vi "Main IU.vi"() -> ()   [LabVIEW 2019]
uses:
  <vilib>/Analysis/baseanly.llb/Mean (DBL).vi
  <vilib>/Analysis/NI_AALBase.lvlib
panel:
  out "Numeric":dbl
  in  "RESET 2":bool
  in  "Tiempo 2":dbl
  in  "Tiempo 1":dbl
  in  "Home":bool
  in  "Aceleración final Motor 2":dbl
  in  "Aceleración final Motor 1":dbl
  in  "Velocidad final Motor 2":dbl
  in  "Velocidad final Motor 1":dbl
  out "String":string
  in  "GO 2":bool
  in  "Aceleración inicial Motor 2":dbl
  in  "Aceleración inicial Motor 1":dbl
  in  "Velocidad inicial Motor 2":dbl
  in  "Velocidad inicial Motor 1":dbl
  in  "RESET 1":bool
  in  "Trayectoria":bool
  in  "GO":bool
  in  "Posición final Motor 2":dbl
  in  "MOTORES INDEPENDIENTES":bool
  in  "Tab Control":enum32{"Motor 1", "Motor 2"}(tab)
  out "Waveform Chart 6":waveform(dbl)[](graph)
  out "Waveform Chart 5":waveform(dbl)[](graph)
  out "Hall 1":bool
  out "Posición":waveform(dbl)[](graph)
  out "Hall 2":bool
  out "Waveform Chart 4":waveform(dbl)[](graph)
  out "Waveform Chart 3":waveform(dbl)[](graph)
  out "Hall 2":bool
  out "Waveform Chart 2":waveform(dbl)[](graph)
  out "Hall1":bool
  out "Saving Data":bool
  in  "Record Button":bool
  in  "Filename":path=path "test.lvm"
  in  "Stop UI and RT":bool
  in  "Stop UI":bool
  in  "Posición final motor 1":dbl
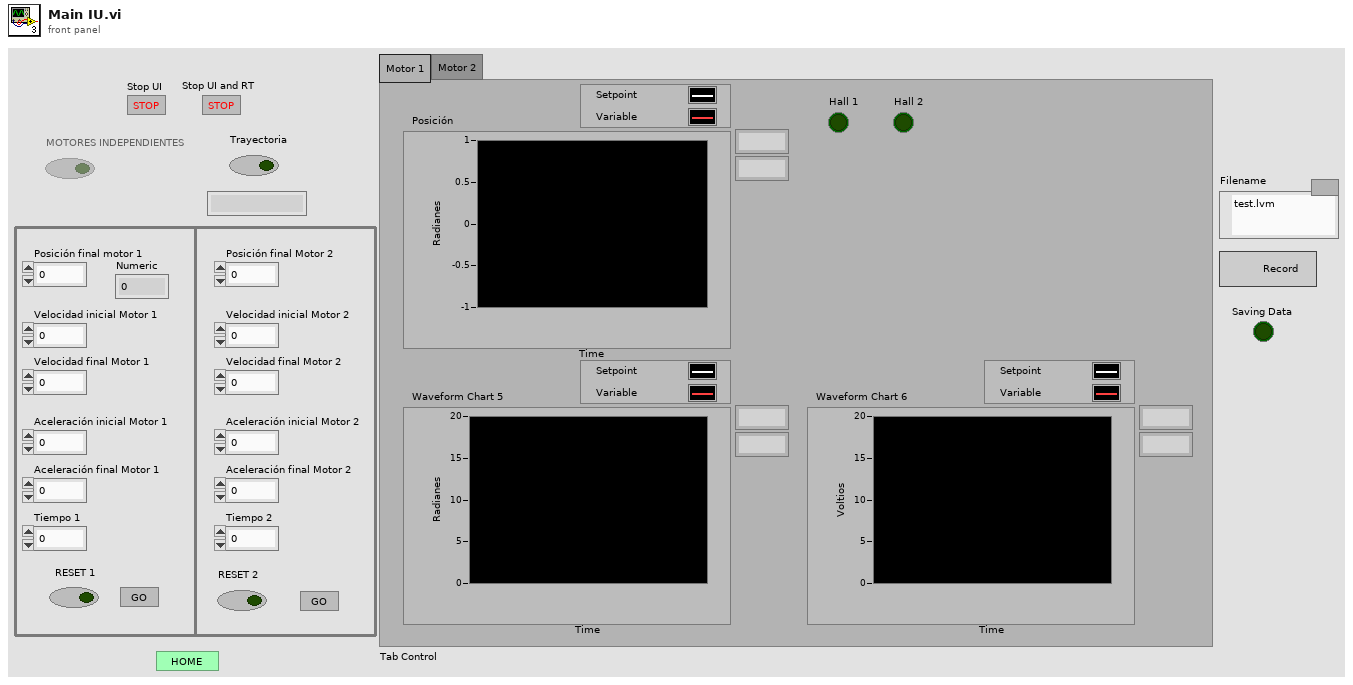
[diagram p1: front panel]
types:
  T1 = cluster{"Double":dbl, "dbl Scaled Value":dbl, "Output":dbl, "seconds since 1Jan1904":timestamp}
  T2 = cluster{"Double":dbl, "dbl Scaled Value":dbl, "Output":dbl, "seconds since 1Jan1904":timestamp}[]
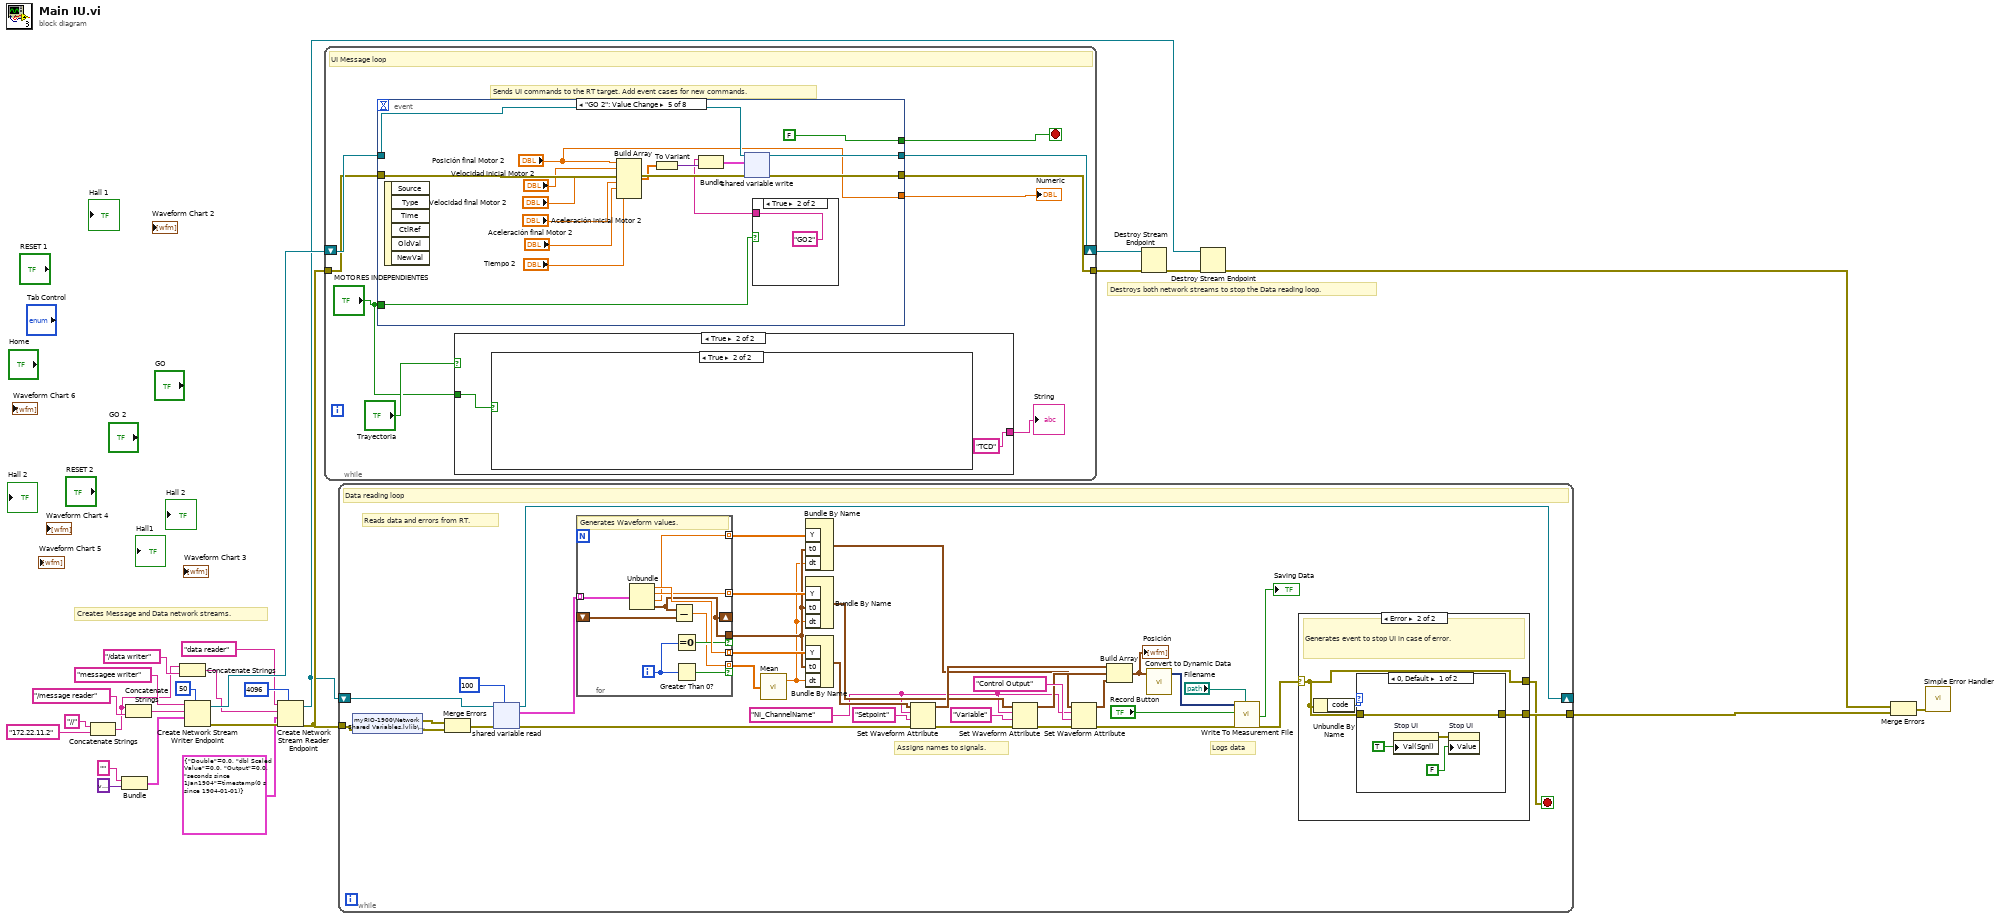
[diagram p0: block diagram]
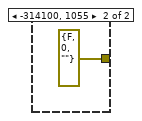
[diagram p3: hidden frame]
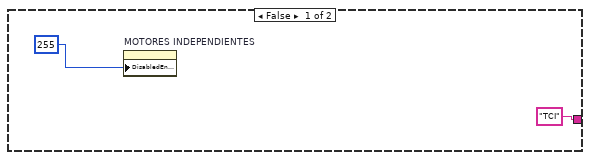
[diagram p4: hidden frame]
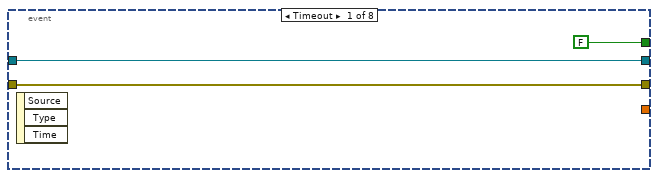
[diagram p6: hidden frame]
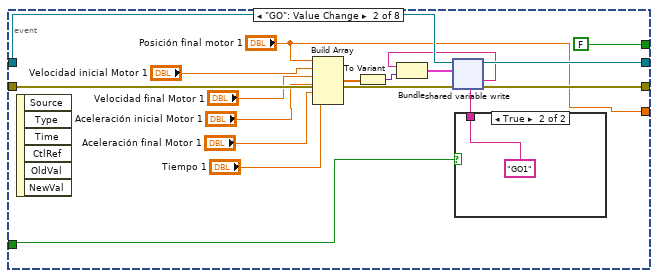
[diagram p7: hidden frame]
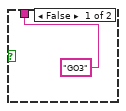
[diagram p8: hidden frame]
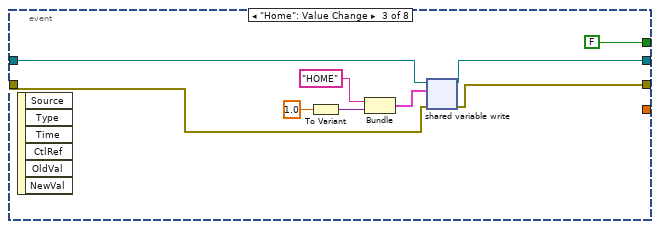
[diagram p9: hidden frame]
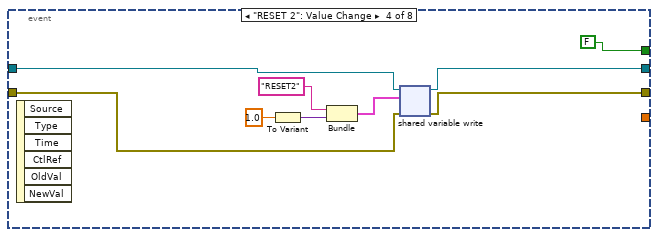
[diagram p10: hidden frame]
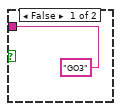
[diagram p11: hidden frame]
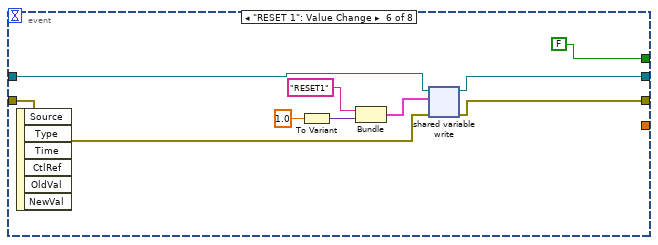
[diagram p12: hidden frame]
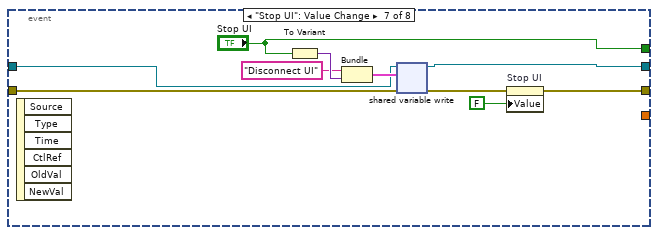
[diagram p13: hidden frame]
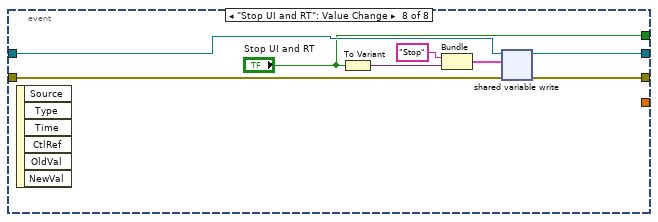
[diagram p14: hidden frame]
diagram:
  # "Destroys both network streams to stop the Data reading loop."
  # "Creates Message and Data network streams."
  n1 = Concatenate Strings("//", "172.22.11.2" ("myRIO IP")) -> (w1:string)
  n2 = Bundle("", variant) -> (w25:cluster{string, variant})  [unwired: 1 in]
  n3 = Concatenate Strings(w1, "/message reader") -> (w2:string)
  n4 = Concatenate Strings(w1, "/data writer") -> (w16:string)
  n5 = Create Network Stream Writer Endpoint(7:50 ("writer buffer size"), 9:w25, 10:w2, 11:"messagee writer" ("writer name")) -> (0:w13:errorcluster, 3:w19:refnum<k21>)  [unwired: 3 in]
  n6 = Create Network Stream Reader Endpoint(7:4096 ("reader buffer size"), 8:w13, 9:T1 {"Double"=0.0, "dbl Scaled Value"=0.0, "Output"=0.0, "seconds since 1Jan1904"=timestamp(0 s since 1904-01-01)} ("Data"), 10:w16, 11:"data reader" ("reader name")) -> (0:w12:errorcluster, 3:w5:refnum<k21>)  [unwired: 2 in]
  n7 = while {
    tunnel: w12 -> [w33]
    shift-right: [w32] -> w7
    shift-left: w19 -> [w34]
    tunnel: [w31] -> w8
    stop <- w30 stop-if-true
    # "Sends UI commands to the RT target. Add event cases for new commands."
    # "UI Message loop"
    n8 = event shown="[4] \"GO 2\": Value Change" {
      selector: _ -> [_ _ _ _ _ _ _ _]
      dyn-events: _ -> [_ _ _ _ _ _ _ _]
      timeout: _ -> [_ _ _ _ _ _ _ _]
      tunnel: w34 -> [w41 w57 w65 w71 w90 w99 w111 w116]
      tunnel: w33 -> [w39 w56 w62 w70 w88 w97 w107 w119]
      tunnel: [w41 w53 w64 w72 w91 w100 w110 w117] -> w32
      tunnel: [w39 w52 w63 w73 w89 w98 w105 w118] -> w31
      tunnel: [FALSE ("Stop UI and RT") FALSE ("Stop UI and RT") FALSE FALSE ("Stop UI and RT") FALSE ("Stop UI and RT") FALSE ("Stop UI and RT") "Stop UI" "Stop UI and RT"] -> w30
      tunnel: "MOTORES INDEPENDIENTES" -> [_ w47 _ _ w80 _ _ _]
      tunnel: [_ "Posición final motor 1" _ _ "Posición final Motor 2" _ _ _] -> w28
      event Timeout {
        n9 = event-data() -> ()  [unwired: 1 in, 3 out]
      }
      event "GO": Value Change {
        n10 = event-data() -> ()  [unwired: 1 in, 6 out]
        n11 = Build Array("Posición final motor 1", "Velocidad inicial Motor 1", "Velocidad final Motor 1", "Aceleración inicial Motor 1", "Aceleración final Motor 1", "Tiempo 1") -> (w49:dbl[])
        n12 = To Variant(anything=w49) -> (Variant=w55:variant)
        n13 = case shown="True" w47 {
          tunnel: ["GO3" ("writer name") "GO1" ("writer name")] -> w50
          frame False {
          }
          frame True {
          }
        }
        n14 = Bundle("writer name"=w50, "Variant"=w55) -> (w54:cluster{"writer name":string, "Variant":variant})  [unwired: 1 in]
        n15 = shared-variable-write(w57, w56, w54) -> (w53:refnum<k21>, w52:errorcluster)  [unwired: 1 in, 1 out]
      }
      event "Home": Value Change {
        n16 = event-data() -> ()  [unwired: 1 in, 6 out]
        n17 = To Variant(anything=1.0) -> (Variant=w68:variant)
        n18 = Bundle("writer name"="HOME", "Variant"=w68) -> (w66:cluster{"writer name":string, "Variant":variant})  [unwired: 1 in]
        n19 = shared-variable-write(w65, w62, w66) -> (w64:refnum<k21>, w63:errorcluster)  [unwired: 1 in, 1 out]
      }
      event "RESET 2": Value Change {
        n20 = event-data() -> ()  [unwired: 1 in, 6 out]
        n21 = To Variant(anything=1.0) -> (Variant=w76:variant)
        n22 = Bundle("writer name"="RESET2", "Variant"=w76) -> (w77:cluster{"writer name":string, "Variant":variant})  [unwired: 1 in]
        n23 = shared-variable-write(w71, w70, w77) -> (w72:refnum<k21>, w73:errorcluster)  [unwired: 1 in, 1 out]
      }
      event "GO 2": Value Change {
        n24 = event-data() -> ()  [unwired: 1 in, 6 out]
        n25 = Build Array("Posición final Motor 2", "Velocidad inicial Motor 2", "Velocidad final Motor 2", "Aceleración inicial Motor 2", "Aceleración final Motor 2", "Tiempo 2") -> (w86:dbl[])
        n26 = To Variant(anything=w86) -> (Variant=w93:variant)
        n27 = case shown="True" w80 {
          tunnel: ["GO3" ("writer name") "GO2" ("writer name")] -> w79
          frame False {
          }
          frame True {
          }
        }
        n28 = Bundle("writer name"=w79, "Variant"=w93) -> (w92:cluster{"writer name":string, "Variant":variant})  [unwired: 1 in]
        n29 = shared-variable-write(w90, w88, w92) -> (w91:refnum<k21>, w89:errorcluster)  [unwired: 1 in, 1 out]
      }
      event "RESET 1": Value Change {
        n30 = event-data() -> ()  [unwired: 1 in, 6 out]
        n31 = To Variant(anything=1.0) -> (Variant=w103:variant)
        n32 = Bundle("writer name"="RESET1", "Variant"=w103) -> (w104:cluster{"writer name":string, "Variant":variant})  [unwired: 1 in]
        n33 = shared-variable-write(w99, w97, w104) -> (w100:refnum<k21>, w98:errorcluster)  [unwired: 1 in, 1 out]
      }
      event "Stop UI": Value Change {
        n34 = event-data() -> ()  [unwired: 1 in, 6 out]
        n35 = To Variant(anything="Stop UI") -> (Variant=w114:variant)
        n36 = Bundle("writer name"="Disconnect UI", "Variant"=w114) -> (w113:cluster{"writer name":string, "Variant":variant})  [unwired: 1 in]
        n37 = shared-variable-write(w111, w107, w113) -> (w110:refnum<k21>, w106:errorcluster)  [unwired: 1 in, 1 out]
        n38 = property on="Stop UI" class="Bool (strict)"(error in=w106, "Value"=FALSE ("Stop UI and RT")) -> (error out=w105:errorcluster)  [unwired: 1 in, 1 out]
      }
      event "Stop UI and RT": Value Change {
        n39 = event-data() -> ()  [unwired: 1 in, 6 out]
        n40 = To Variant(anything="Stop UI and RT") -> (Variant=w122:variant)
        n41 = Bundle("writer name"="Stop", "Variant"=w122) -> (w121:cluster{"writer name":string, "Variant":variant})  [unwired: 1 in]
        n42 = shared-variable-write(w116, w119, w121) -> (w117:refnum<k21>, w118:errorcluster)  [unwired: 1 in, 1 out]
      }
    }
    "Numeric" <- w28
    n43 = case shown="True" "Trayectoria" {
      tunnel: ["TCI" "TCD"] -> w29
      tunnel: "MOTORES INDEPENDIENTES" -> [_ w37]
      frame False {
        n44 = property on="MOTORES INDEPENDIENTES" class="Bool (strict)"("DisabledEnum"=255) -> ()  [unwired: 2 in, 2 out]
      }
      frame True {
        n45 = case shown="True" w37 {
          frame False {
          }
          frame True {
          }
        }
      }
    }
    "String" <- w29
  }
  n46 = while {
    tunnel: w12 -> [w126]
    shift-right: [w139] -> _
    shift-left: w5 -> [w158]
    tunnel: [w125] -> w9
    stop <- w124 stop-if-true
    w130 = "NI_ChannelName" ("name")
    # "Logs data"
    # "Assigns names to signals."
    # "Reads data and errors from RT."
    # "Data reading loop"
    n47 = shared-variable "myRIO-1900\\Network Shared Variables.lvlib\\error IO"(error in=w126) -> (w129:errorcluster, error out=w128:errorcluster)
    n48 = Merge Errors(w129, w128) -> (w127:errorcluster)
    n49 = shared-variable-read(w158, w127, 100 ("# elements")) -> (w139:refnum<k21>, w147:errorcluster, w157:T2)  [unwired: 1 in, 1 out]
    n50 = for {
      tunnel: w157 -> [w177] mode=indexing
      tunnel: [w176] -> w156 mode=indexing
      tunnel: [w175] -> w155 mode=indexing
      tunnel: [w174] -> w154 mode=indexing
      tunnel: [w172] -> w153 if=w173
      shift-right: [w172] -> _
      shift-left: _ -> [w171]
      tunnel: [w170] -> w131 mode=indexing if=w168
      i -> [w169]
      # "Generates Waveform values."
      n51 = Unbundle(w177) -> ("Double"=w176:dbl, "dbl Scaled Value"=w175:dbl, "Output"=w174:dbl, "seconds since 1Jan1904"=w172:timestamp)
      n52 = Subtract(x=w172, y=w171) -> (x-y=w170:dbl)
      n53 = Equal To 0?(x=w169) -> (x = 0?=w173:bool)
      n54 = Greater Than 0?(x=w169) -> (x > 0?=w168:bool)
    }
    n55 = call-poly <vilib>:"Mean.vi"("X"=w131) -> ("mean"=w152:dbl)  [unwired: 1 out]
    n56 = Bundle By Name("Y"=w154, "t0"=w153, "dt"=w152) -> (w141:waveform(dbl))  [unwired: 1 in]
    n57 = Bundle By Name("Y"=w155, "t0"=w153, "dt"=w152) -> (w142:waveform(dbl))  [unwired: 1 in]
    n58 = Bundle By Name("Y"=w156, "t0"=w153, "dt"=w152) -> (w151:waveform(dbl))  [unwired: 1 in]
    n59 = Set Waveform Attribute(4:w147, 5:"Setpoint" ("name"), 6:w130, 7:w151) -> (0:w146:errorcluster, 3:w144:waveform(dbl))  [unwired: 1 out]
    n60 = Set Waveform Attribute(4:w146, 5:"Variable" ("name"), 6:w130, 7:w142) -> (0:w145:errorcluster, 3:w143:waveform(dbl))  [unwired: 1 out]
    n61 = Set Waveform Attribute(4:w145, 5:"Control Output" ("name"), 6:w130, 7:w141) -> (0:w138:errorcluster, 3:w140:waveform(dbl))  [unwired: 1 out]
    n62 = Build Array(w144, w143, w140) -> (w137:waveform(dbl)[])
    "Posición" <- w137
    n63 = call "Convert to Dynamic Data"("Array of Waveforms"=w137) -> ("Dynamic Data Type"=w136:dynamicdata)  [unwired: 3 in]
    n64 = call "Write To Measurement File"("Signals"=w136, "Enable"="Record Button", "error in (no error)"=w138, "Filename"="Filename") -> ("Saving Data"=→"Saving Data":bool, "error out"=w132:errorcluster)  [unwired: 13 in, 1 out]
    n65 = case shown="Error" w132 {
      selector: w132 -> [w159 w160]
      tunnel: [w159 w161] -> w125
      tunnel: [w159 w160] -> w124
      frame No Error {
        # "No action required."
      }
      frame Error {
        # "Generates event to stop UI in case of error."
        n66 = Unbundle By Name(w160) -> ("code"=w162:i32)
        n67 = case shown="0, Default" w162 {
          tunnel: [w165 errorcluster {"status"=FALSE, "code"=0, "source"=""} ("error IO")] -> w161
          tunnel: w160 -> [w165 _]
          frame 0, Default {
            n68 = property on="Stop UI" class="Bool (strict)"("Val(Sgnl)"=TRUE ("Stop UI and RT")) -> (error out=w164:errorcluster)  [unwired: 2 in, 1 out]
            n69 = property on="Stop UI" class="Bool (strict)"(error in=w164, "Value"=FALSE ("Stop UI")) -> ()  [unwired: 1 in, 2 out]
          }
          frame -314100, 1055 {
          }
        }
      }
    }
  }
  n70 = Destroy Stream Endpoint(8:w8, 11:w7) -> (0:w6:errorcluster)
  n71 = Destroy Stream Endpoint(8:w6, 11:w5) -> (0:w4:errorcluster)
  n72 = Merge Errors(w4, w9) -> (w10:errorcluster)
  n73 = call <vilib>:"Simple Error Handler.vi"("error in (no error)"=w10) -> ()  [unwired: 4 in, 5 out]
